vi "Read Outputs to system.vi"(8 "error in":errorcluster, 11 "ThreePhasePLL runtime in":refnum<class "ThreePhasePLL runtime.lvclass">) -> (0 "error out":errorcluster, 2 "Outputs to system":T1, 3 "ThreePhasePLL runtime out":refnum<class "ThreePhasePLL runtime.lvclass">)   [LabVIEW 2017, in "ThreePhasePLL runtime.lvclass"]
uses:
  ThreePhasePLL runtime.lvclass
  configuration/output data indices.ctl
  ThreePhasePLL runtime.lvclass/ThreePhasePLL runtime.ctl
  configuration/ThreePhasePLL configuration.lvclass
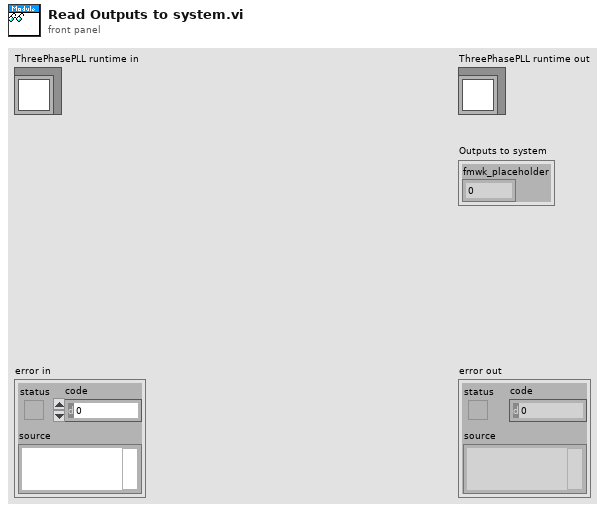
[diagram p1: front panel]
types:
  T1 = typedef "ThreePhasePLL configuration.lvclass/output data indices.ctl" = cluster{"fmwk_placeholder":i32}
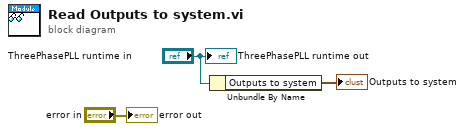
[diagram p0: block diagram]
diagram:
  n1 = Unbundle By Name("ThreePhasePLL runtime in") -> ("Outputs to system"=→"Outputs to system":T1)
  "error out" <- "error in"
  "ThreePhasePLL runtime out" <- "ThreePhasePLL runtime in"
